vi "Parse Status Line.vi"(11 "Headers w/ status line":string) -> (0 "HTTP Version":string, 1 "HTTP Headers":string, 2 "Status String":string, 3 "status code":u16, 5 "Status Line":string)   [LabVIEW 2020, in "httpClient.lvlib" / "httpClient.lvclass"]
uses:
  httpClient.lvclass
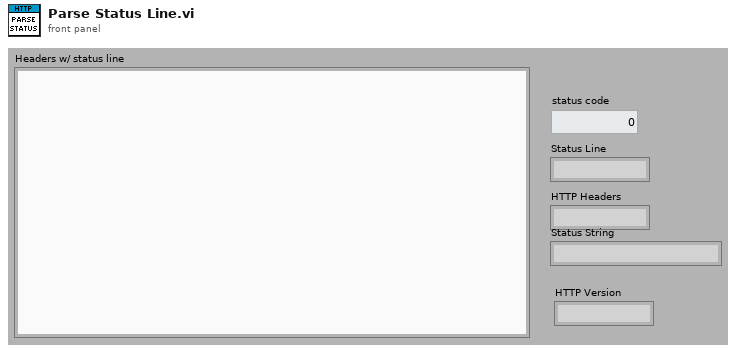
[diagram p1: front panel]
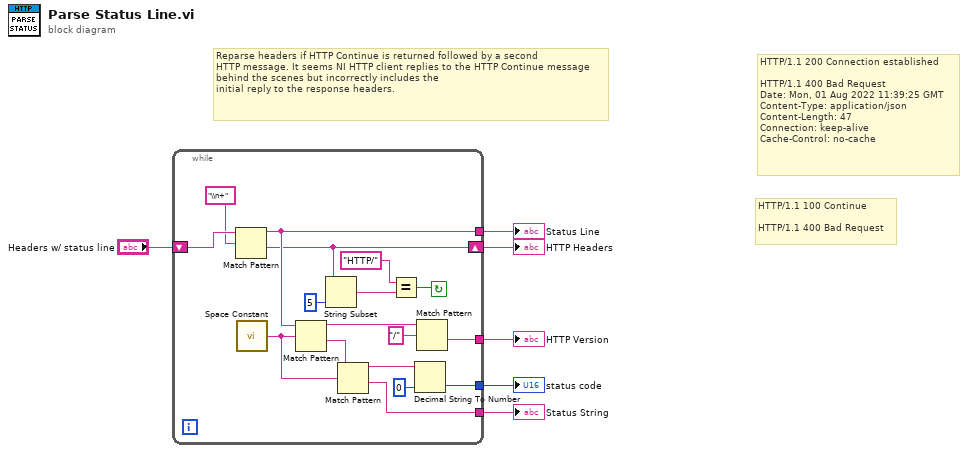
[diagram p0: block diagram]
diagram:
  # "Reparse headers if HTTP Continue is returned followed by a second\nHTTP message. It seems NI HTTP client replies to the HTTP Continue message behind the scenes but incorrectly includes the\ninitial reply to the response headers."
  # "HTTP/1.1 200 Connection established\n\nHTTP/1.1 400 Bad Request\nDate: Mon, 01 Aug 2022 11:39:25 GMT\nContent-Type: application/json\nContent-Length: 47\nConnection: keep-alive\nCache-Control: no-cache"
  # "HTTP/1.1 100 Continue\n\nHTTP/1.1 400 Bad Request"
  n1 = while {
    shift-right: [w8] -> w1
    shift-left: "Headers w/ status line" -> [w23]
    tunnel: [w22] -> w5
    tunnel: [w20] -> w4
    tunnel: [w14] -> w2
    tunnel: [w18] -> w3
    stop <- w9 continue-if-true
    n2 = Match Pattern(string=w23, regular expression="\\n+") -> (before substring=w22:string, after substring=w8:string)  [unwired: 1 in, 2 out]
    n3 = call <vilib>:"Space Constant.vi"() -> ("String"=w19:string)
    n4 = Match Pattern(string=w22, regular expression=w19) -> (before substring=w10:string, after substring=w11:string)  [unwired: 1 in, 2 out]
    n5 = String Subset(string=w8, length (rest)=5 ("length (rest)")) -> (substring=w12:string)  [unwired: 1 in]
    n6 = Match Pattern(string=w11, regular expression=w19) -> (before substring=w16:string, after substring=w18:string)  [unwired: 1 in, 2 out]
    n7 = Equal?(x="HTTP/", y=w12) -> (x = y?=w9:bool)
    n8 = Decimal String To Number(string=w16, default (0L)=u16 0 ("default (0 I32)")) -> (number=w14:u16)  [unwired: 1 in, 1 out]
    n9 = Match Pattern(string=w10, regular expression="/") -> (after substring=w20:string)  [unwired: 1 in, 3 out]
  }
  "Status Line" <- w5
  "HTTP Headers" <- w1
  "HTTP Version" <- w4
  "Status String" <- w3
  "status code" <- w2
